vi "Read Scalar Data.vi"(8 "error in (no error)":errorcluster, 10 "Values":dbl[](array[numeric]), 11 "Cluster":T1 {"Data Type" format="%.0x"}) -> (0 "error out":errorcluster, 2 "Values":dbl[](array[numeric]), 3 "Cluster":T1 {"Data Type" format="%.0x"})   [LabVIEW 2015, in "FPGA Addon Engine.lvlib"]
uses:
  FPGA Addon Engine.lvlib
  Types/Register Settings.ctl
  Shared/Data Type.ctl
  Shared/Scalar Type.ctl
  <vilib>/rvi/errors/niLvFpgaAdjustHostInterfaceError.vi
  <vilib>/Utility/error.llb/Error Cluster From Error Code.vi
  <vilib>/rvi/interface/nirviReadWriteControl/nirviReadWriteControl.xnode
  NiFpgaLv.dll
  <vilib>/rvi/interface/Simulation/niFpgaSimulationCallBeginRW.vi
  Shared/FPGA Addon Shared.lvlib
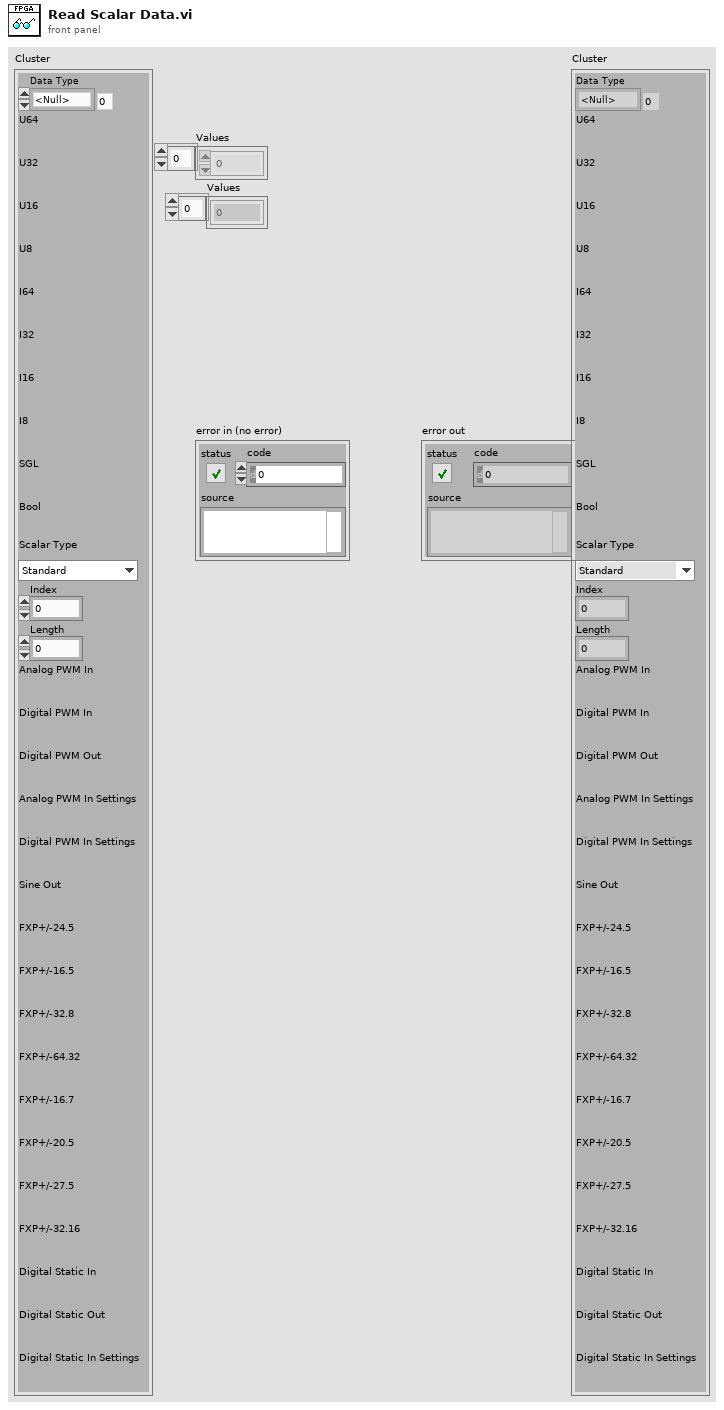
[diagram p1: front panel]
types:
  T1 = typedef "FPGA Addon Engine.lvlib/Register Settings.ctl" = cluster{"Data Type":T2, "U64":refnum<k20>, "U32":refnum<k20>, "U16":refnum<k20>, "U8":refnum<k20>, "I64":refnum<k20>, "I32":refnum<k20>, "I16":refnum<k20>, "I8":refnum<k20>, "SGL":refnum<k20>, "Bool":refnum<k20>, "Scalar Type":T3, "Index":i32, "Length":i32, "Analog PWM In":refnum<k20>, "Digital PWM In":refnum<k20>, "Digital PWM Out":refnum<k20>, "Analog PWM In Settings":refnum<k20>, "Digital PWM In Settings":refnum<k20>, "Sine Out":refnum<k20>, "FXP+/-24.5":refnum<k20>, "FXP+/-16.5":refnum<k20>, "FXP+/-32.8":refnum<k20>, "FXP+/-64.32":refnum<k20>, "FXP+/-16.7":refnum<k20>, "FXP+/-20.5":refnum<k20>, "FXP+/-27.5":refnum<k20>, "FXP+/-32.16":refnum<k20>, "Digital Static In":refnum<k20>, "Digital Static Out":refnum<k20>, "Digital Static In Settings":refnum<k20>}
  T2 = typedef "FPGA Addon Shared.lvlib/Data Type.ctl" = enum8{"<Null>", "I8", "I16", "I32", "I64", "U8", "U16", "U32", "U64", "SGL", "Boolean", "Analog PWM In Settings", "Analog PWM In", "Digital PWM In Settings", "Digital PWM In", "Digital PWM Out", "Sine Out", "FXP+/-24.5", "FXP+/-16.5", "FXP+/-32.8", "FXP+/-64.32", "FXP+/-16.7", "FXP+/-20.5", "FXP+/-27.5", "FXP+/-32.16", "Digital Static In", "Digital Static Out", "Digital Static In Settings"}
  T3 = typedef "FPGA Addon Shared.lvlib/Scalar Type.ctl" = enum16{"Standard", "Bitpacked"}
  T4 = cluster{"ACTIVE TICKS":u32, "INACTIVE TICKS":u32, "ACQ TICKS":u32, "ACTIVE VOLTAGE":fxp<+/-,32,8>, "INACTIVE VOLTAGE":fxp<+/-,32,8>}
  T5 = cluster{"ACTIVE TICKS":u32, "INACTIVE TICKS":u32, "ACQ TICKS":u32}
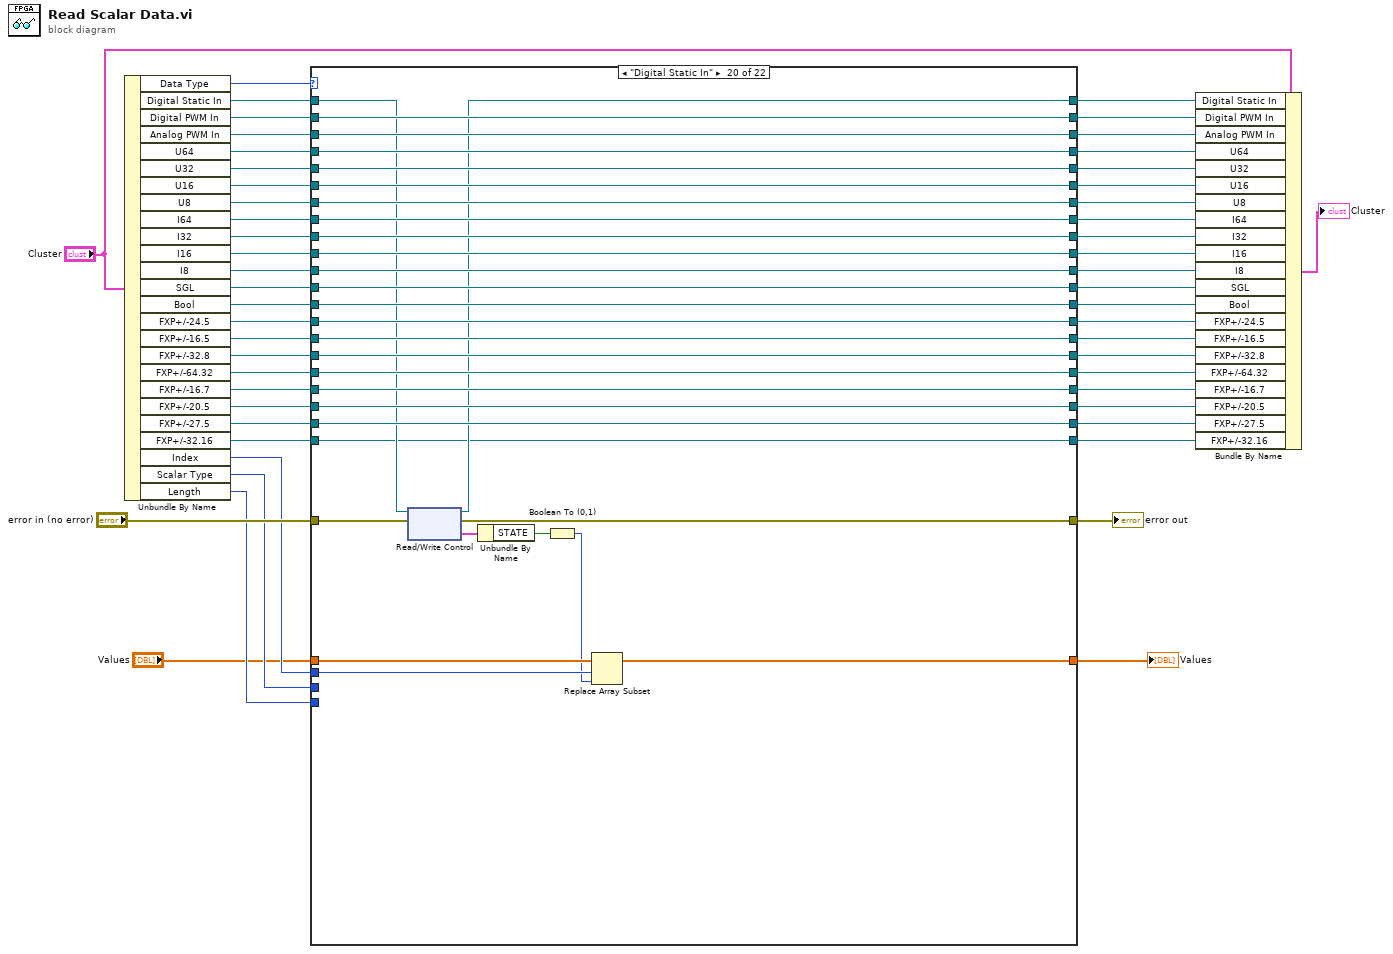
[diagram p0: block diagram]
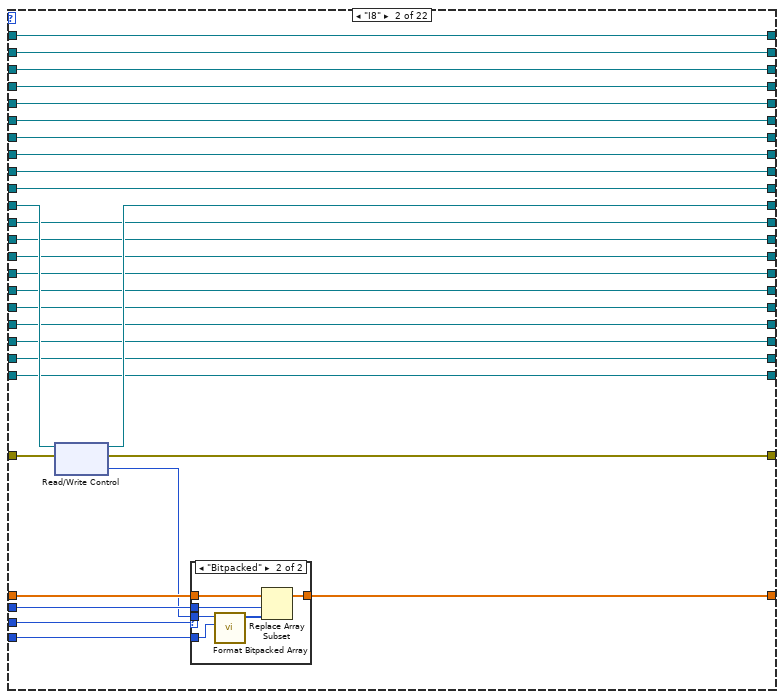
[diagram p3: hidden frame]
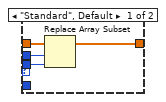
[diagram p4: hidden frame]
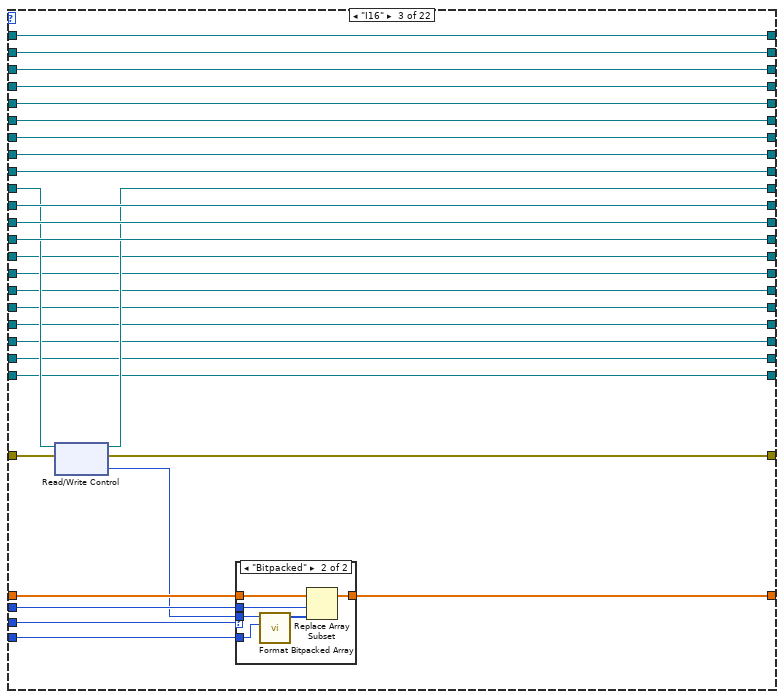
[diagram p5: hidden frame]
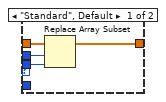
[diagram p6: hidden frame]
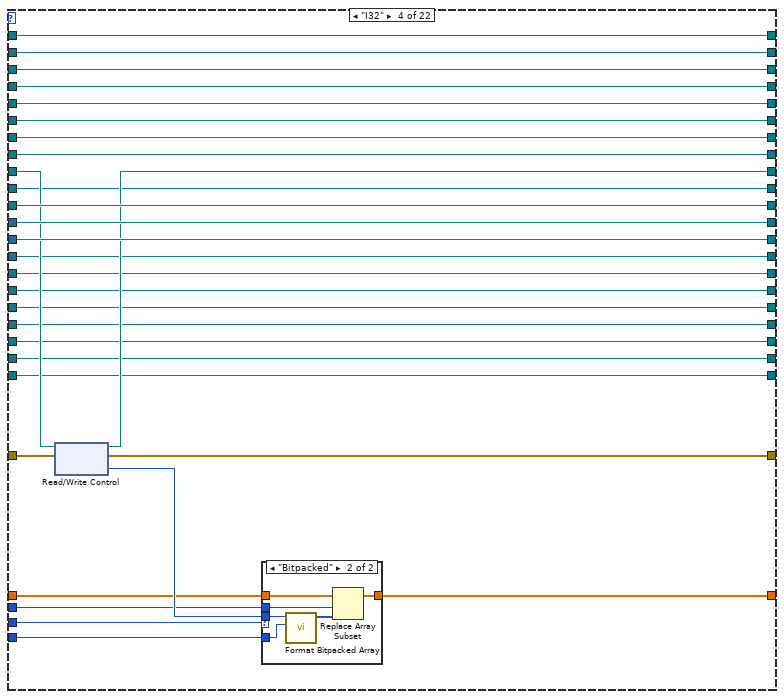
[diagram p7: hidden frame]
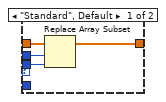
[diagram p8: hidden frame]
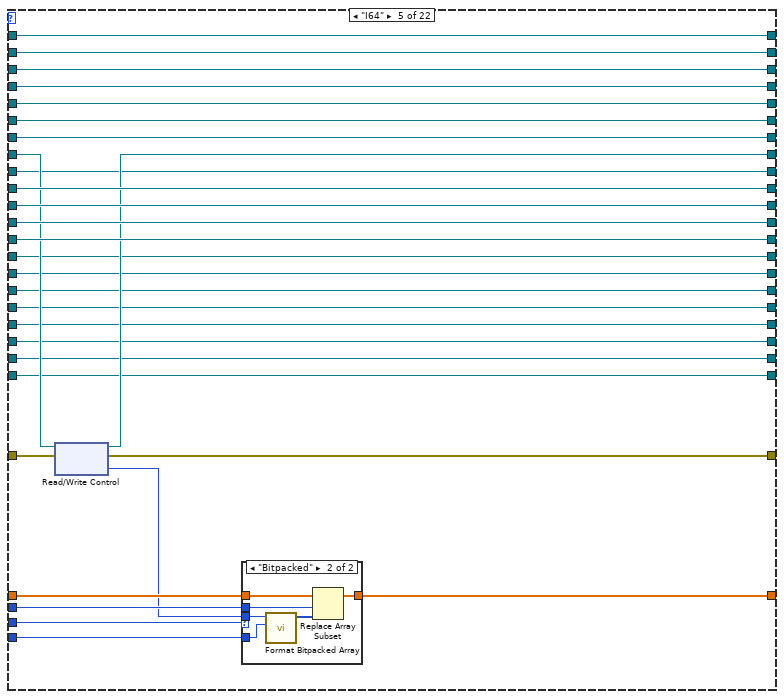
[diagram p9: hidden frame]
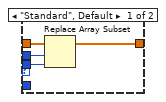
[diagram p10: hidden frame]
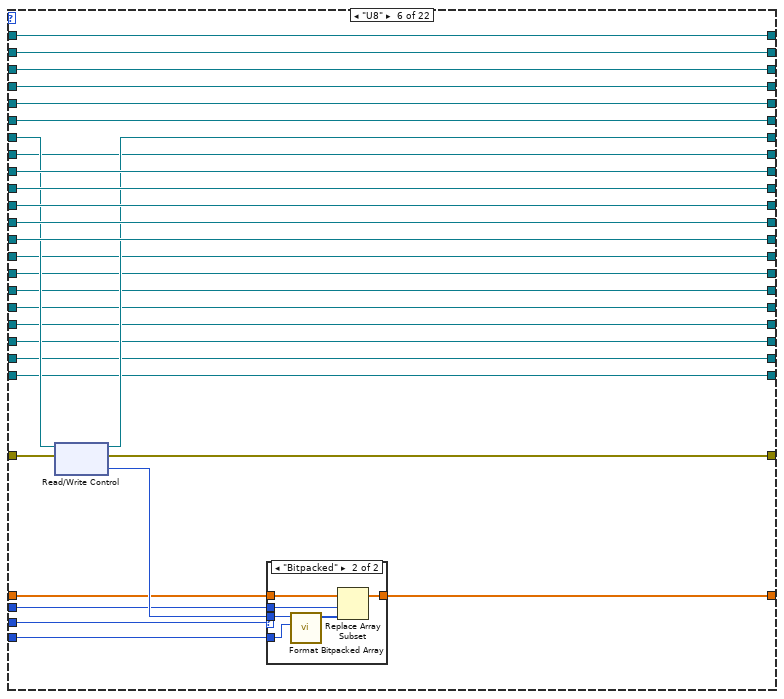
[diagram p11: hidden frame]
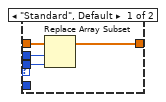
[diagram p12: hidden frame]
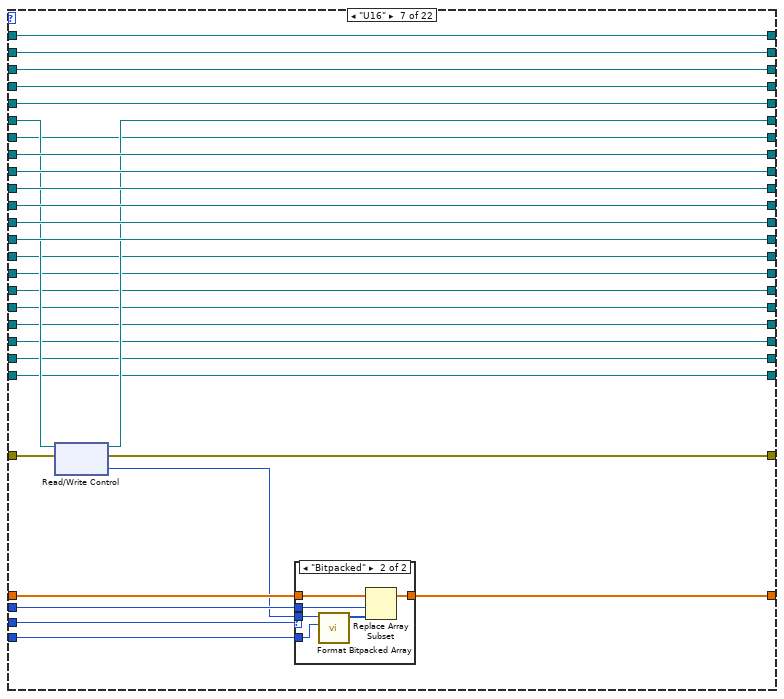
[diagram p13: hidden frame]
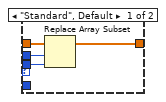
[diagram p14: hidden frame]
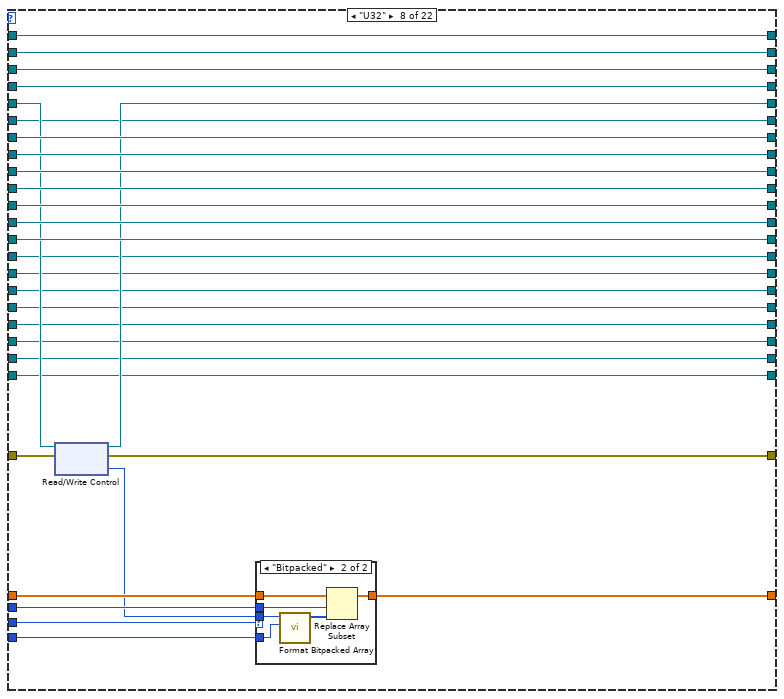
[diagram p15: hidden frame]
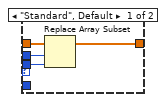
[diagram p16: hidden frame]
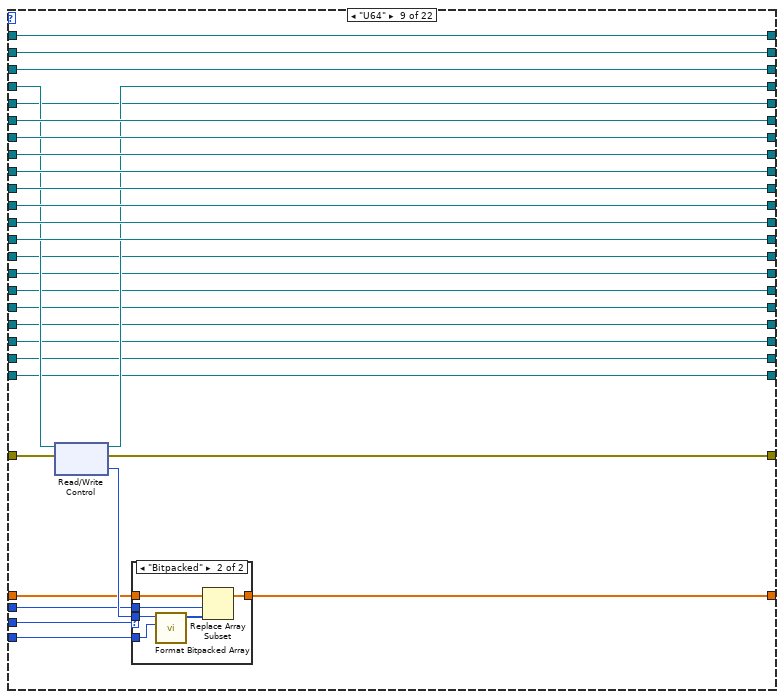
[diagram p17: hidden frame]
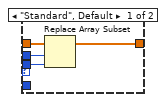
[diagram p18: hidden frame]
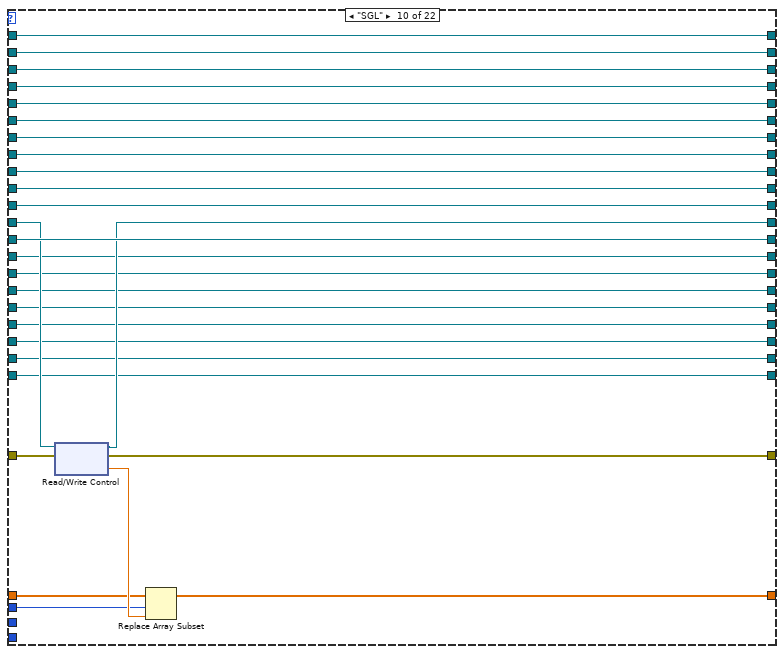
[diagram p19: hidden frame]
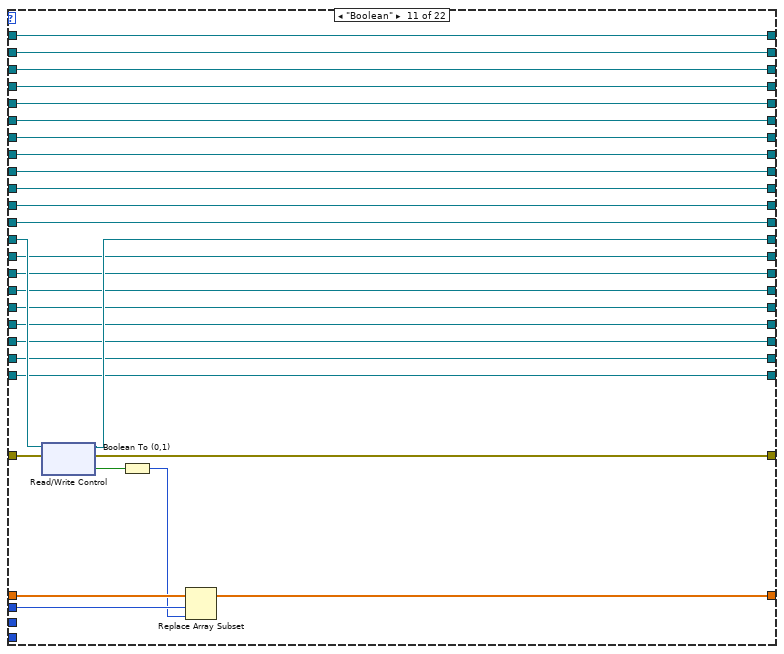
[diagram p20: hidden frame]
diagram:
  n1 = Unbundle By Name("Cluster") -> ("Data Type"=w3:T2, "Digital Static In"=w2:refnum<k20>, "Digital PWM In"=w21:refnum<k20>, "Analog PWM In"=w22:refnum<k20>, "U64"=w30:refnum<k20>, "U32"=w32:refnum<k20>, "U16"=w34:refnum<k20>, "U8"=w36:refnum<k20>, "I64"=w38:refnum<k20>, "I32"=w40:refnum<k20>, "I16"=w42:refnum<k20>, "I8"=w52:refnum<k20>, "SGL"=w46:refnum<k20>, "Bool"=w45:refnum<k20>, "FXP+/-24.5"=w19:refnum<k20>, "FXP+/-16.5"=w16:refnum<k20>, "FXP+/-32.8"=w15:refnum<k20>, "FXP+/-64.32"=w12:refnum<k20>, "FXP+/-16.7"=w10:refnum<k20>, "FXP+/-20.5"=w8:refnum<k20>, "FXP+/-27.5"=w7:refnum<k20>, "FXP+/-32.16"=w4:refnum<k20>, "Index"=w26:i32, "Scalar Type"=w27:T3, "Length"=w28:i32)
  n2 = case shown="\"Digital Static In\"" w3 {
    tunnel: w52 -> [w73 w105 w135 w176 w217 w258 w299 w340 w381 w420 w450 w478 w506 w534 w562 w590 w618 w646 w674 w704 w747 w800]
    tunnel: "error in (no error)" -> [w65 w104 w145 w185 w225 w265 w305 w345 w385 w423 w452 w480 w508 w536 w564 w592 w620 w648 w676 w706 w744 w797]
    tunnel: [w65 w103 w144 w184 w224 w264 w304 w344 w384 w422 w451 w479 w507 w535 w563 w591 w619 w647 w675 w705 w743 w796] -> w50
    tunnel: [w73 w102 w135 w176 w217 w258 w299 w340 w381 w420 w450 w478 w506 w534 w562 w590 w618 w646 w674 w704 w747 w800] -> w48
    tunnel: [w74 w101 w143 w183 w223 w263 w303 w343 w383 w411 w440 w470 w498 w526 w554 w582 w610 w638 w666 w696 w746 w799] -> w47
    tunnel: w46 -> [w74 w101 w143 w183 w223 w263 w303 w343 w383 w413 w440 w470 w498 w526 w554 w582 w610 w638 w666 w696 w746 w799]
    tunnel: w45 -> [w75 w100 w142 w182 w222 w262 w302 w342 w382 w421 w442 w463 w492 w520 w548 w576 w604 w632 w660 w690 w745 w798]
    tunnel: [w75 w100 w142 w182 w222 w262 w302 w342 w382 w421 w441 w463 w492 w520 w548 w576 w604 w632 w660 w690 w745 w798] -> w44
    tunnel: [w72 w99 w133 w173 w216 w257 w298 w339 w380 w419 w449 w477 w505 w533 w561 w589 w617 w645 w673 w703 w748 w801] -> w43
    tunnel: w42 -> [w72 w99 w134 w173 w216 w257 w298 w339 w380 w419 w449 w477 w505 w533 w561 w589 w617 w645 w673 w703 w748 w801]
    tunnel: [w71 w98 w141 w174 w213 w256 w297 w338 w379 w418 w448 w476 w504 w532 w560 w588 w616 w644 w672 w702 w749 w802] -> w41
    tunnel: w40 -> [w71 w98 w141 w175 w213 w256 w297 w338 w379 w418 w448 w476 w504 w532 w560 w588 w616 w644 w672 w702 w749 w802]
    tunnel: [w70 w97 w140 w181 w214 w253 w296 w337 w378 w417 w447 w475 w503 w531 w559 w587 w615 w643 w671 w701 w750 w803] -> w39
    tunnel: w38 -> [w70 w97 w140 w181 w215 w253 w296 w337 w378 w417 w447 w475 w503 w531 w559 w587 w615 w643 w671 w701 w750 w803]
    tunnel: [w69 w96 w139 w180 w221 w254 w293 w336 w377 w416 w446 w474 w502 w530 w558 w586 w614 w642 w670 w700 w751 w804] -> w37
    tunnel: w36 -> [w69 w96 w139 w180 w221 w255 w293 w336 w377 w416 w446 w474 w502 w530 w558 w586 w614 w642 w670 w700 w751 w804]
    tunnel: [w68 w95 w138 w179 w220 w261 w294 w333 w376 w415 w445 w473 w501 w529 w557 w585 w613 w641 w669 w699 w752 w805] -> w35
    tunnel: w34 -> [w68 w95 w138 w179 w220 w261 w295 w333 w376 w415 w445 w473 w501 w529 w557 w585 w613 w641 w669 w699 w752 w805]
    tunnel: [w67 w94 w137 w178 w219 w260 w301 w334 w373 w414 w444 w472 w500 w528 w556 w584 w612 w640 w668 w698 w753 w806] -> w33
    tunnel: w32 -> [w67 w94 w137 w178 w219 w260 w301 w335 w373 w414 w444 w472 w500 w528 w556 w584 w612 w640 w668 w698 w753 w806]
    tunnel: [w66 w93 w136 w177 w218 w259 w300 w341 w374 w412 w443 w471 w499 w527 w555 w583 w611 w639 w667 w697 w754 w807] -> w31
    tunnel: w30 -> [w66 w93 w136 w177 w218 w259 w300 w341 w375 w412 w443 w471 w499 w527 w555 w583 w611 w639 w667 w697 w754 w807]
    tunnel: w28 -> [_ w89 w129 w167 w209 w249 w292 w328 w369 _ _ _ _ _ _ _ _ _ _ _ _ _]
    tunnel: w27 -> [_ w90 w130 w168 w210 w248 w291 w329 w370 _ _ _ _ _ _ _ _ _ _ _ _ _]
    tunnel: w26 -> [_ w91 w131 w171 w211 w250 w290 w330 w371 w409 w438 w469 w497 w525 w553 w581 w609 w637 w665 w695 w726 w779]
    tunnel: "Values" -> [w64 w92 w132 w170 w212 w251 w289 w332 w368 w408 w437 w468 w496 w524 w552 w580 w608 w636 w664 w694 w728 w781]
    tunnel: [w64 w87 w127 w169 w207 w247 w288 w331 w367 w407 w435 w467 w495 w523 w551 w579 w607 w635 w663 w693 w727 w780] -> w24
    tunnel: [w63 w85 w125 w165 w205 w245 w285 w325 w365 w405 w433 w465 w493 w521 w549 w577 w605 w633 w661 w691 w741 w777] -> w23
    tunnel: w22 -> [w63 w85 w125 w165 w205 w245 w285 w325 w365 w405 w433 w465 w493 w521 w549 w577 w605 w633 w661 w691 w742 w777]
    tunnel: w21 -> [w62 w86 w126 w166 w206 w246 w286 w326 w366 w406 w434 w466 w494 w522 w550 w578 w606 w634 w662 w692 w755 w776]
    tunnel: [w62 w86 w126 w166 w206 w246 w286 w326 w366 w406 w434 w466 w494 w522 w550 w578 w606 w634 w662 w692 w755 w775] -> w20
    tunnel: w19 -> [w61 w84 w124 w164 w204 w244 w284 w324 w364 w404 w432 w464 w486 w517 w546 w574 w602 w630 w658 w688 w715 w769]
    tunnel: [w61 w84 w124 w164 w204 w244 w284 w324 w364 w404 w432 w462 w486 w517 w546 w574 w602 w630 w658 w688 w715 w769] -> w18
    tunnel: [w60 w83 w123 w163 w203 w243 w283 w323 w363 w403 w431 w460 w487 w516 w545 w573 w601 w629 w657 w687 w714 w768] -> w17
    tunnel: w16 -> [w60 w83 w123 w163 w203 w243 w283 w323 w363 w403 w431 w460 w488 w516 w545 w573 w601 w629 w657 w687 w714 w768]
    tunnel: w15 -> [w59 w82 w122 w162 w202 w242 w282 w322 w362 w402 w430 w459 w490 w515 w544 w572 w600 w628 w656 w686 w713 w767]
    tunnel: [w59 w82 w122 w162 w202 w242 w282 w322 w362 w402 w430 w459 w490 w514 w544 w572 w600 w628 w656 w686 w713 w767] -> w14
    tunnel: [w58 w81 w121 w161 w201 w241 w281 w321 w361 w401 w429 w458 w489 w518 w542 w571 w599 w627 w655 w685 w712 w766] -> w13
    tunnel: w12 -> [w58 w81 w121 w161 w201 w241 w281 w321 w361 w401 w429 w458 w489 w518 w543 w571 w599 w627 w655 w685 w712 w766]
    tunnel: [w57 w80 w120 w160 w200 w240 w280 w320 w360 w400 w428 w457 w485 w513 w541 w569 w596 w626 w654 w684 w711 w765] -> w11
    tunnel: w10 -> [w57 w80 w120 w160 w200 w240 w280 w320 w360 w400 w428 w457 w485 w513 w541 w570 w596 w626 w654 w684 w711 w765]
    tunnel: [w56 w79 w119 w159 w199 w239 w279 w319 w359 w399 w427 w456 w484 w512 w540 w568 w598 w624 w653 w683 w710 w764] -> w9
    tunnel: w8 -> [w56 w79 w119 w159 w199 w239 w279 w319 w359 w399 w427 w456 w484 w512 w540 w568 w597 w624 w653 w683 w710 w764]
    tunnel: w7 -> [w55 w78 w118 w158 w198 w238 w278 w318 w358 w398 w426 w455 w483 w511 w539 w567 w595 w625 w652 w682 w709 w763]
    tunnel: [w55 w78 w118 w158 w198 w238 w278 w318 w358 w398 w426 w455 w483 w511 w539 w567 w595 w623 w652 w682 w709 w763] -> w6
    tunnel: [w54 w77 w117 w157 w197 w237 w277 w317 w357 w397 w425 w454 w482 w510 w538 w566 w594 w622 w650 w677 w708 w762] -> w5
    tunnel: w4 -> [w54 w77 w117 w157 w197 w237 w277 w317 w357 w397 w425 w454 w482 w510 w538 w566 w594 w622 w651 w677 w708 w762]
    tunnel: w2 -> [w53 w76 w116 w156 w196 w236 w276 w316 w356 w396 w424 w453 w481 w509 w537 w565 w593 w621 w649 w681 w707 w761]
    tunnel: [w53 w76 w116 w156 w196 w236 w276 w316 w356 w396 w424 w453 w481 w509 w537 w565 w593 w621 w649 w679 w707 w761] -> w1
    frame "<Null>", Default {
    }
    frame "I8" {
      n3 = xnode "Read/Write Control"("FPGA VI Reference In"=w105, "error in"=w104) -> ("FPGA VI Reference Out"=w102:refnum<k20>, "error out"=w103:errorcluster, "Value"=w88:i8)
      n4 = case shown="\"Bitpacked\"" w90 {
        tunnel: w92 -> [w109 w113]
        tunnel: [w108 w112] -> w87
        tunnel: w88 -> [w107 w115]
        tunnel: w91 -> [w106 w110]
        tunnel: w89 -> [_ w114]
        frame "Standard", Default {
          n5 = Replace Array Subset(array=w109, new element=w107, index=w106) -> (w108:dbl[])
        }
        frame "Bitpacked" {
          n6 = call "Format Bitpacked Array.vi"("Length"=w114, "Value"=w115) -> ("Array"=w111:i16[])  [unwired: 9 in]
          n7 = Replace Array Subset(array=w113, new element=w111, index=w110) -> (w112:dbl[])
        }
      }
    }
    frame "I16" {
      n8 = xnode "Read/Write Control"("FPGA VI Reference In"=w134, "error in"=w145) -> ("FPGA VI Reference Out"=w133:refnum<k20>, "error out"=w144:errorcluster, "Value"=w128:i16)
      n9 = case shown="\"Bitpacked\"" w130 {
        tunnel: w132 -> [w149 w153]
        tunnel: [w148 w152] -> w127
        tunnel: w128 -> [w147 w155]
        tunnel: w131 -> [w146 w150]
        tunnel: w129 -> [_ w154]
        frame "Standard", Default {
          n10 = Replace Array Subset(array=w149, new element=w147, index=w146) -> (w148:dbl[])
        }
        frame "Bitpacked" {
          n11 = call "Format Bitpacked Array.vi"("Length"=w154, "Value"=w155) -> ("Array"=w151:i16[])  [unwired: 9 in]
          n12 = Replace Array Subset(array=w153, new element=w151, index=w150) -> (w152:dbl[])
        }
      }
    }
    frame "I32" {
      n13 = xnode "Read/Write Control"("FPGA VI Reference In"=w175, "error in"=w185) -> ("FPGA VI Reference Out"=w174:refnum<k20>, "error out"=w184:errorcluster, "Value"=w172:i32)
      n14 = case shown="\"Bitpacked\"" w168 {
        tunnel: w170 -> [w189 w193]
        tunnel: [w188 w192] -> w169
        tunnel: w172 -> [w187 w195]
        tunnel: w171 -> [w186 w190]
        tunnel: w167 -> [_ w194]
        frame "Standard", Default {
          n15 = Replace Array Subset(array=w189, new element=w187, index=w186) -> (w188:dbl[])
        }
        frame "Bitpacked" {
          n16 = call "Format Bitpacked Array.vi"("Length"=w194, "Value"=w195) -> ("Array"=w191:i16[])  [unwired: 9 in]
          n17 = Replace Array Subset(array=w193, new element=w191, index=w190) -> (w192:dbl[])
        }
      }
    }
    frame "I64" {
      n18 = xnode "Read/Write Control"("FPGA VI Reference In"=w215, "error in"=w225) -> ("FPGA VI Reference Out"=w214:refnum<k20>, "error out"=w224:errorcluster, "Value"=w208:i64)
      n19 = case shown="\"Bitpacked\"" w210 {
        tunnel: w212 -> [w229 w233]
        tunnel: [w228 w232] -> w207
        tunnel: w208 -> [w227 w235]
        tunnel: w211 -> [w226 w230]
        tunnel: w209 -> [_ w234]
        frame "Standard", Default {
          n20 = Replace Array Subset(array=w229, new element=w227, index=w226) -> (w228:dbl[])
        }
        frame "Bitpacked" {
          n21 = call "Format Bitpacked Array.vi"("Length"=w234, "Value"=w235) -> ("Array"=w231:i16[])  [unwired: 9 in]
          n22 = Replace Array Subset(array=w233, new element=w231, index=w230) -> (w232:dbl[])
        }
      }
    }
    frame "U8" {
      n23 = xnode "Read/Write Control"("FPGA VI Reference In"=w255, "error in"=w265) -> ("FPGA VI Reference Out"=w254:refnum<k20>, "error out"=w264:errorcluster, "Value"=w252:u8)
      n24 = case shown="\"Bitpacked\"" w248 {
        tunnel: w251 -> [w269 w273]
        tunnel: [w268 w272] -> w247
        tunnel: w252 -> [w267 w275]
        tunnel: w250 -> [w266 w270]
        tunnel: w249 -> [_ w274]
        frame "Standard", Default {
          n25 = Replace Array Subset(array=w269, new element=w267, index=w266) -> (w268:dbl[])
        }
        frame "Bitpacked" {
          n26 = call "Format Bitpacked Array.vi"("Length"=w274, "Value"=w275) -> ("Array"=w271:i16[])  [unwired: 9 in]
          n27 = Replace Array Subset(array=w273, new element=w271, index=w270) -> (w272:dbl[])
        }
      }
    }
    frame "U16" {
      n28 = xnode "Read/Write Control"("FPGA VI Reference In"=w295, "error in"=w305) -> ("FPGA VI Reference Out"=w294:refnum<k20>, "error out"=w304:errorcluster, "Value"=w287:u16)
      n29 = case shown="\"Bitpacked\"" w291 {
        tunnel: w289 -> [w309 w313]
        tunnel: [w308 w312] -> w288
        tunnel: w287 -> [w307 w315]
        tunnel: w290 -> [w306 w310]
        tunnel: w292 -> [_ w314]
        frame "Standard", Default {
          n30 = Replace Array Subset(array=w309, new element=w307, index=w306) -> (w308:dbl[])
        }
        frame "Bitpacked" {
          n31 = call "Format Bitpacked Array.vi"("Length"=w314, "Value"=w315) -> ("Array"=w311:i16[])  [unwired: 9 in]
          n32 = Replace Array Subset(array=w313, new element=w311, index=w310) -> (w312:dbl[])
        }
      }
    }
    frame "U32" {
      n33 = xnode "Read/Write Control"("FPGA VI Reference In"=w335, "error in"=w345) -> ("FPGA VI Reference Out"=w334:refnum<k20>, "error out"=w344:errorcluster, "Value"=w327:u32)
      n34 = case shown="\"Bitpacked\"" w329 {
        tunnel: w332 -> [w349 w353]
        tunnel: [w348 w352] -> w331
        tunnel: w327 -> [w347 w355]
        tunnel: w330 -> [w346 w350]
        tunnel: w328 -> [_ w354]
        frame "Standard", Default {
          n35 = Replace Array Subset(array=w349, new element=w347, index=w346) -> (w348:dbl[])
        }
        frame "Bitpacked" {
          n36 = call "Format Bitpacked Array.vi"("Length"=w354, "Value"=w355) -> ("Array"=w351:i16[])  [unwired: 9 in]
          n37 = Replace Array Subset(array=w353, new element=w351, index=w350) -> (w352:dbl[])
        }
      }
    }
    frame "U64" {
      n38 = xnode "Read/Write Control"("FPGA VI Reference In"=w375, "error in"=w385) -> ("FPGA VI Reference Out"=w374:refnum<k20>, "error out"=w384:errorcluster, "Value"=w372:u64)
      n39 = case shown="\"Bitpacked\"" w370 {
        tunnel: w368 -> [w389 w393]
        tunnel: [w388 w392] -> w367
        tunnel: w372 -> [w387 w395]
        tunnel: w371 -> [w386 w390]
        tunnel: w369 -> [_ w394]
        frame "Standard", Default {
          n40 = Replace Array Subset(array=w389, new element=w387, index=w386) -> (w388:dbl[])
        }
        frame "Bitpacked" {
          n41 = call "Format Bitpacked Array.vi"("Length"=w394, "Value"=w395) -> ("Array"=w391:i16[])  [unwired: 9 in]
          n42 = Replace Array Subset(array=w393, new element=w391, index=w390) -> (w392:dbl[])
        }
      }
    }
    frame "SGL" {
      n43 = xnode "Read/Write Control"("FPGA VI Reference In"=w413, "error in"=w423) -> ("FPGA VI Reference Out"=w411:refnum<k20>, "error out"=w422:errorcluster, "Value"=w410:sgl)
      n44 = Replace Array Subset(array=w408, new element=w410, index=w409) -> (w407:dbl[])
    }
    frame "Boolean" {
      n45 = xnode "Read/Write Control"("FPGA VI Reference In"=w442, "error in"=w452) -> ("FPGA VI Reference Out"=w441:refnum<k20>, "error out"=w451:errorcluster, "Value"=w439:bool)
      n46 = Boolean To (0,1)(Boolean=w439) -> (0, 1=w436:i16)
      n47 = Replace Array Subset(array=w437, new element=w436, index=w438) -> (w435:dbl[])
    }
    frame "FXP+/-24.5" {
      n48 = xnode "Read/Write Control"("FPGA VI Reference In"=w464, "error in"=w480) -> ("FPGA VI Reference Out"=w462:refnum<k20>, "error out"=w479:errorcluster, "Value"=w461:fxp<+/-,24,5>)
      n49 = Replace Array Subset(array=w468, new element=w461, index=w469) -> (w467:dbl[])
    }
    frame "FXP+/-16.5" {
      n50 = xnode "Read/Write Control"("FPGA VI Reference In"=w488, "error in"=w508) -> ("FPGA VI Reference Out"=w487:refnum<k20>, "error out"=w507:errorcluster, "Value"=w491:fxp<+/-,16,5>)
      n51 = Replace Array Subset(array=w496, new element=w491, index=w497) -> (w495:dbl[])
    }
    frame "FXP+/-32.8" {
      n52 = xnode "Read/Write Control"("FPGA VI Reference In"=w515, "error in"=w536) -> ("FPGA VI Reference Out"=w514:refnum<k20>, "error out"=w535:errorcluster, "Value"=w519:fxp<+/-,32,8>)
      n53 = Replace Array Subset(array=w524, new element=w519, index=w525) -> (w523:dbl[])
    }
    frame "FXP+/-64.32" {
      n54 = xnode "Read/Write Control"("FPGA VI Reference In"=w543, "error in"=w564) -> ("FPGA VI Reference Out"=w542:refnum<k20>, "error out"=w563:errorcluster, "Value"=w547:fxp<+/-,64,32>)
      n55 = Replace Array Subset(array=w552, new element=w547, index=w553) -> (w551:dbl[])
    }
    frame "FXP+/-16.7" {
      n56 = xnode "Read/Write Control"("FPGA VI Reference In"=w570, "error in"=w592) -> ("FPGA VI Reference Out"=w569:refnum<k20>, "error out"=w591:errorcluster, "Value"=w575:fxp<+/-,16,7>)
      n57 = Replace Array Subset(array=w580, new element=w575, index=w581) -> (w579:dbl[])
    }
    frame "FXP+/-20.5" {
      n58 = xnode "Read/Write Control"("FPGA VI Reference In"=w597, "error in"=w620) -> ("FPGA VI Reference Out"=w598:refnum<k20>, "error out"=w619:errorcluster, "Value"=w603:fxp<+/-,20,5>)
      n59 = Replace Array Subset(array=w608, new element=w603, index=w609) -> (w607:dbl[])
    }
    frame "FXP+/-27.5" {
      n60 = xnode "Read/Write Control"("FPGA VI Reference In"=w625, "error in"=w648) -> ("FPGA VI Reference Out"=w623:refnum<k20>, "error out"=w647:errorcluster, "Value"=w631:fxp<+/-,27,5>)
      n61 = Replace Array Subset(array=w636, new element=w631, index=w637) -> (w635:dbl[])
    }
    frame "FXP+/-32.16" {
      n62 = xnode "Read/Write Control"("FPGA VI Reference In"=w651, "error in"=w676) -> ("FPGA VI Reference Out"=w650:refnum<k20>, "error out"=w675:errorcluster, "Value"=w659:fxp<+/-,32,16>)
      n63 = Replace Array Subset(array=w664, new element=w659, index=w665) -> (w663:dbl[])
    }
    frame "Digital Static In" {
      n64 = xnode "Read/Write Control"("FPGA VI Reference In"=w681, "error in"=w706) -> ("FPGA VI Reference Out"=w679:refnum<k20>, "error out"=w705:errorcluster, "Value"=w689:cluster{"STATE":bool})
      n65 = Unbundle By Name(w689) -> ("STATE"=w680:bool)
      n66 = Boolean To (0,1)(Boolean=w680) -> (0, 1=w678:i16)
      n67 = Replace Array Subset(array=w694, new element=w678, index=w695) -> (w693:dbl[])
    }
    frame "Analog PWM In" {
      w735 = 2.5000000292152436e-08 ("y")
      n68 = xnode "Read/Write Control"("FPGA VI Reference In"=w742, "error in"=w744) -> ("FPGA VI Reference Out"=w741:refnum<k20>, "error out"=w743:errorcluster, "Value"=w723:T4)
      n69 = Unbundle By Name(w723) -> ("ACTIVE TICKS"=w722:u32, "INACTIVE TICKS"=w721:u32, "ACQ TICKS"=w720:u32, "ACTIVE VOLTAGE"=w719:fxp<+/-,32,8>, "INACTIVE VOLTAGE"=w718:fxp<+/-,32,8>)
      n70 = Add(x=w722, y=w721) -> (x+y=w737:u32)
      n71 = Compound Arithmetic op=MULTIPLY(w737, w720, w735) -> (w738:dbl)
      n72 = Divide(x=w722, y=w737) -> (x/y=w731:dbl)
      n73 = Compound Arithmetic op=MULTIPLY(w722, w720, w735) -> (w736:dbl)
      n74 = Multiply(x=100.0, y=w731) -> (x*y=w730:dbl)
      n75 = Equal?(x=0.0, y=w738) -> (x = y?=w734:bool)
      n76 = Reciprocal(x=w738) -> (1/x=w739:dbl)
      n77 = case shown="False" w734 {
        tunnel: [w756 w760] -> w717
        tunnel: [w757 w760] -> w724
        tunnel: [w759 w760] -> w716
        tunnel: w738 -> [w759 _]
        tunnel: [w758 w760] -> w729
        tunnel: w736 -> [w758 _]
        tunnel: w730 -> [w757 _]
        tunnel: w739 -> [w756 _]
        tunnel: 0.0 ("x") -> [_ w760]
        frame False {
        }
        frame True {
        }
      }
      n78 = Build Array(w717, w716, w724, w729, w719, w718) -> (w725:dbl[])
      n79 = Replace Array Subset(array=w728, new element=w725, index=w726) -> (w727:dbl[])
    }
    frame "Digital PWM In" {
      w790 = 2.5000000292152436e-08 ("y")
      n80 = xnode "Read/Write Control"("FPGA VI Reference In"=w776, "error in"=w797) -> ("FPGA VI Reference Out"=w775:refnum<k20>, "error out"=w796:errorcluster, "Value"=w783:T5)
      n81 = Unbundle By Name(w783) -> ("ACTIVE TICKS"=w773:u32, "INACTIVE TICKS"=w772:u32, "ACQ TICKS"=w786:u32)
      n82 = Add(x=w773, y=w772) -> (x+y=w792:u32)
      n83 = Compound Arithmetic op=MULTIPLY(w792, w786, w790) -> (w793:dbl)
      n84 = Divide(x=w773, y=w792) -> (x/y=w785:dbl)
      n85 = Compound Arithmetic op=MULTIPLY(w773, w786, w790) -> (w791:dbl)
      n86 = Multiply(x=100.0, y=w785) -> (x*y=w784:dbl)
      n87 = Equal?(x=0.0, y=w793) -> (x = y?=w789:bool)
      n88 = Reciprocal(x=w793) -> (1/x=w794:dbl)
      n89 = case shown="False" w789 {
        tunnel: [w808 w812] -> w771
        tunnel: [w809 w812] -> w774
        tunnel: [w811 w812] -> w770
        tunnel: w793 -> [w811 _]
        tunnel: [w810 w812] -> w782
        tunnel: w791 -> [w810 _]
        tunnel: w784 -> [w809 _]
        tunnel: w794 -> [w808 _]
        tunnel: 0.0 ("x") -> [_ w812]
        frame False {
        }
        frame True {
        }
      }
      n90 = Build Array(w771, w770, w774, w782) -> (w778:dbl[])
      n91 = Replace Array Subset(array=w781, new element=w778, index=w779) -> (w780:dbl[])
    }
  }
  "error out" <- w50
  "Values" <- w24
  n92 = Bundle By Name(cluster="Cluster", "Digital Static In"=w1, "Digital PWM In"=w20, "Analog PWM In"=w23, "U64"=w31, "U32"=w33, "U16"=w35, "U8"=w37, "I64"=w39, "I32"=w41, "I16"=w43, "I8"=w48, "SGL"=w47, "Bool"=w44, "FXP+/-24.5"=w18, "FXP+/-16.5"=w17, "FXP+/-32.8"=w14, "FXP+/-64.32"=w13, "FXP+/-16.7"=w11, "FXP+/-20.5"=w9, "FXP+/-27.5"=w6, "FXP+/-32.16"=w5) -> (→"Cluster":T1)
